vi "serialization tests.vi"() -> ()   [LabVIEW 2013, in "Profibus Module tests.lvlib"]
uses:
  Profibus Module tests.lvlib
  configuration/Profibus Module configuration.lvclass
panel:
  out "channels equal":bool
  out "no error":errorcluster
  out "no error":errorcluster
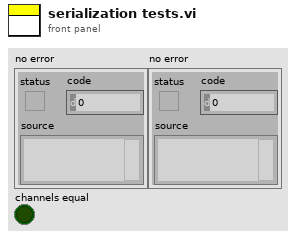
[diagram p1: front panel]
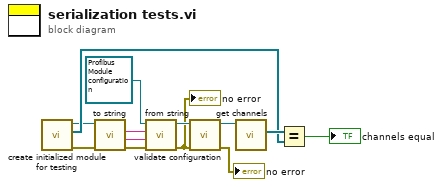
[diagram p0: block diagram]
diagram:
  n1 = call "create initialized module for testing.vi"() -> ("error out"=w1:errorcluster, "1d channels"=w3:refnum<class "Profibus channel.lvclass">[], "Profibus Module configuration out"=w2:refnum<class "Profibus Module configuration.lvclass">)  [unwired: 6 in, 3 out]
  n2 = call-dynamic "to string.vi"("error in"=w1, "Profibus Module configuration in"=w2) -> ("error out"=w13:errorcluster, "data"=w12:string, "version"=w11:string)  [unwired: 6 in, 1 out]
  n3 = call-dynamic "from string.vi"("error in"=w13, "data"=w12, "version"=w11, "Profibus Module configuration in"=refnum<class "Profibus Module configuration.lvclass"> refnum ("tag bus configurable plugin module configuration")) -> ("error out"=w8:errorcluster, "Profibus Module configuration out"=w10:refnum<class "Profibus Module configuration.lvclass">)  [unwired: 6 in]
  "no error" <- w8
  n4 = call-dynamic "validate configuration.vi"("error in"=w8, "Profibus Module configuration in"=w10) -> ("error out"=→"no error":errorcluster, "Profibus Module configuration out"=w5:refnum<class "Profibus Module configuration.lvclass">)  [unwired: 8 in]
  n5 = call-dynamic "get channels.vi"("Profibus Module configuration in"=w5) -> ("channels"=w4:refnum<class "TBM channel.lvclass">[])  [unwired: 9 in, 1 out]
  n6 = Equal?(x=w4, y=w3) -> (x = y?=→"channels equal":bool)
